vi "displayConfigurableElements.vi"(11 "ConfigurationThisComponent in":refnum<class "ConfigurationTestParameters.lvclass">) -> (3 "ConfigurationThisComponent out":refnum<class "ConfigurationTestParameters.lvclass">)   [LabVIEW 2013, in "ConfigurationTestParameters.lvclass"]
uses:
  ConfigurationTestParameters.lvclass
  Configuration/TestParameters.ctl
  Configuration/CycleProfileConfig.ctl
  <userlib>/Common/Log/Config/Log.ctl
  <userlib>/Common/Log/Log.lvlib
panel:
  in  "ctrlRefArrayUsrEvnt":refnum<user-event>
  in  "ConfigTab":enum32{"Test Parameters", "Test Data Log"}(tab)
  in  "TestParameters":T1={"Number of cycles for complete test"=0, "Cycle profile"={"Temperature Setpoint"=[], "Soak Time"=[], "Gain Stabilization Time"=[], "Pause After Step"=[]}, "PGA Gain Coefficients"=[], "Temperature Transition Wait Time"=0.0, "Temperature Settled StDev"=273.15, "Temperature Settling Sample Size"=0, "Bridge Measurement Sample Size"=0} {"Temperature Settling Sample Size" min=1; "Bridge Measurement Sample Size" min=1; "Temperature Settled StDev" min=271.15 max=275.15 format="%.4f"; "PGA Gain Coefficients" max=7; "Temperature Transition Wait Time" min=1.0; "Cycle profile"."Gain Stabilization Time" min=0.0 max=600.0 format="%.1f"; "Cycle profile"."Soak Time" min=0.0 max=600.0 format="%.1f"; "Cycle profile"."Pause After Step" min=0.0 max=600.0 format="%.1f"; "Cycle profile"."Temperature Setpoint" min=233.14999999999998 max=313.15 format="%.1f"; "Number of cycles for complete test" min=1}
  in  "TestDataLog":T3={"Log Directory"=path "", "Log Filename Base"="", "Max records per file"=1000, "Comment"=""} {"Max records per file" min=100 max=1000000}
  # "Gain is 2^gain_coefficient"
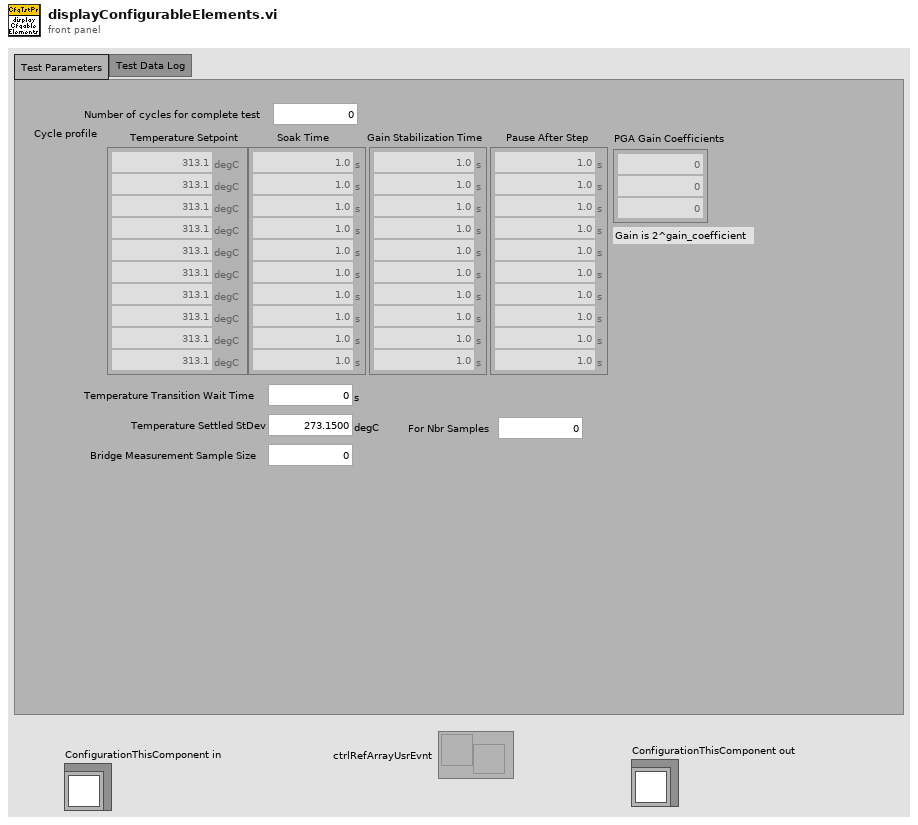
[diagram p1: front panel]
types:
  T1 = typedef "TestParameters.ctl" = cluster{"Number of cycles for complete test":u32, "Cycle profile":T2, "PGA Gain Coefficients":u8[], "Temperature Transition Wait Time":dbl[unit], "Temperature Settled StDev":dbl[unit], "Temperature Settling Sample Size":u16, "Bridge Measurement Sample Size":u16}
  T2 = typedef "CycleProfileConfig.ctl" = cluster{"Temperature Setpoint":dbl[unit][], "Soak Time":dbl[unit][], "Gain Stabilization Time":dbl[unit][], "Pause After Step":dbl[unit][]}
  T3 = typedef "Log.lvlib/Log.ctl" = cluster{"Log Directory":path, "Log Filename Base":string, "Max records per file":u32, "Comment":string}
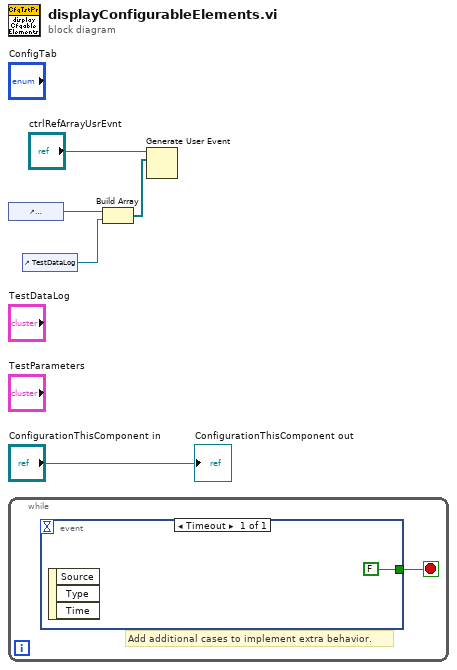
[diagram p0: block diagram]
diagram:
  n1 = control-ref of="TestParameters"() -> (w3:refnum<vi>)
  n2 = while {
    stop <- w6 stop-if-true
    # "Add additional cases to implement extra behavior."
    n3 = event shown="[0] Timeout" {
      selector: _ -> [_]
      dyn-events: _ -> [_]
      timeout: _ -> [_]
      tunnel: [FALSE] -> w6
      event Timeout {
        n4 = event-data() -> ()  [unwired: 1 in, 3 out]
      }
    }
  }
  n5 = control-ref of="TestDataLog"() -> (w1:refnum<vi>)
  n6 = Build Array(w3, w1) -> (w2:refnum<vi>[])
  n7 = Generate User Event(user event="ctrlRefArrayUsrEvnt", event data cluster=w2) -> ()  [unwired: 2 in, 2 out]
  "ConfigurationThisComponent out" <- "ConfigurationThisComponent in"
